vi "epxMAUpdate.vi"(8 "expFactor":i16=-8, 10 "update":i16, 11 "carryIn":fxp<+/-,22,16>) -> (3 "carryOut":fxp<+/-,22,16>)   [LabVIEW 2016]
uses:
  <vilib>/rvi/FXPMathLib/FxpSub/XNode/nifxpmath_Sub.xnode
  <vilib>/rvi/FXPMathLib/FxpAdd/XNode/nifxpmath_Add.xnode
  <vilib>/rvi/FXPMathLib/sim/FxpSim.dll
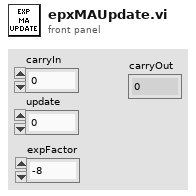
[diagram p1: front panel]
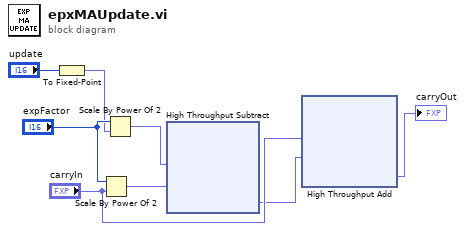
[diagram p0: block diagram]
diagram:
  n1 = To Fixed-Point(number="update") -> (fixed-point=w4:fxp<+/-,22,16>)  [unwired: 1 in]
  n2 = Scale By Power Of 2(n="expFactor", x="carryIn") -> (x*2^n=w6:fxp<+/-,22,16>)
  n3 = Scale By Power Of 2(n="expFactor", x=w4) -> (x*2^n=w7:fxp<+/-,22,16>)
  n4 = xnode "High Throughput Subtract"("x"=w7, "y"=w6) -> ("x-y"=w2:fxp<+/-,22,16>)
  n5 = xnode "High Throughput Add"("x"="carryIn", "y"=w2) -> ("x+y"=→"carryOut":fxp<+/-,22,16>)
